vi "HXG2_FlowAir_STD51.vi"(0 "1\" Nozzle":bool, 1 "0.75\" Nozzle":bool, 2 "2.5inWC Sensor?":bool, 5 "1.25\" Nozzle":bool, 7 "1.5\" Nozzle":bool, 9 "Nozzle in Td °F":dbl, 11 "error in (no error)":errorcluster, 12 "Nozzle in %RH":dbl, 13 "Nozzle DP inWC":dbl, 14 "Pbarometric psi":dbl) -> (3 "CFM Nozzle":dbl, 4 "MaxSCFM":dbl, 6 "MinSCFM":dbl, 8 "Mdot (lbm/hr)":dbl, 10 "Rho per ASHRAE":dbl, 15 "error out":errorcluster)   [LabVIEW 2012]
doc: "This VI will calculate volumetric flow and provide the max and min flows that can be achieved with a particular nozzle combination."
panel:
  out "Pws Eqn":dbl
  out "Patm (psia)":dbl
  out "PabsUUT (inWC)":dbl
  out "All Psychrometric Calcs":sgl[](array[numeric])
  out "Pw":sgl
  out "W":sgl
  out "v":sgl
  out "ALPHA":sgl format="%#.3f"
  out "Ce 1":dbl[](array[numeric])
  out "Ce":dbl[](array[numeric])
  out "Re":dbl[](array[numeric])
  out "Y":sgl
  out "mu":sgl format="%#.6f"
  out "output variable":i16
  out "Pws":dbl
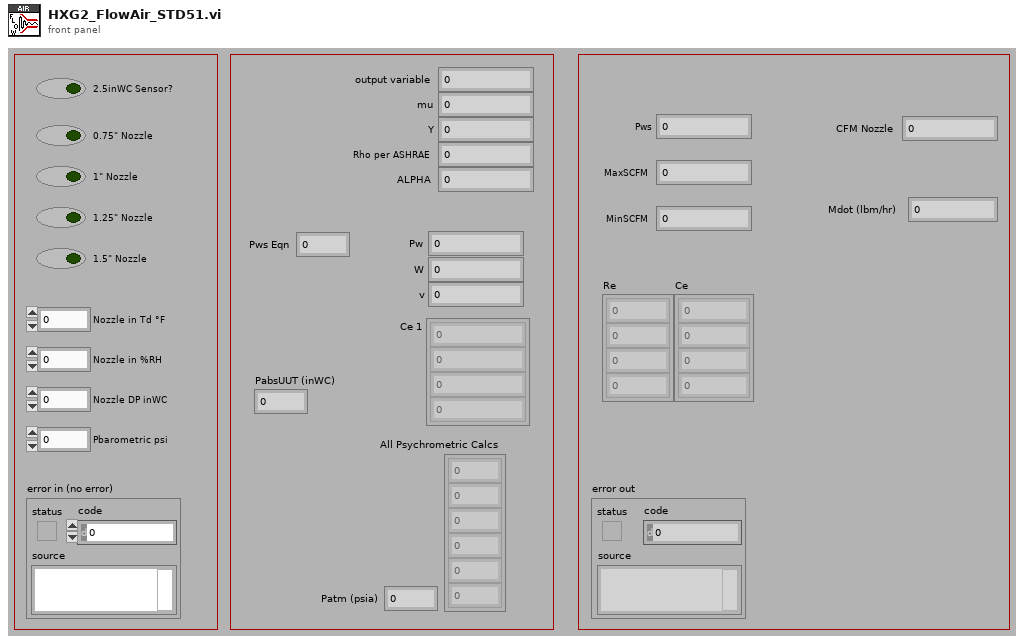
[diagram p1: front panel]
types:
  T1 = enum16{"Initial Values", "Closed Nozzle", "Iterate", "Recalc Re", "Done"}
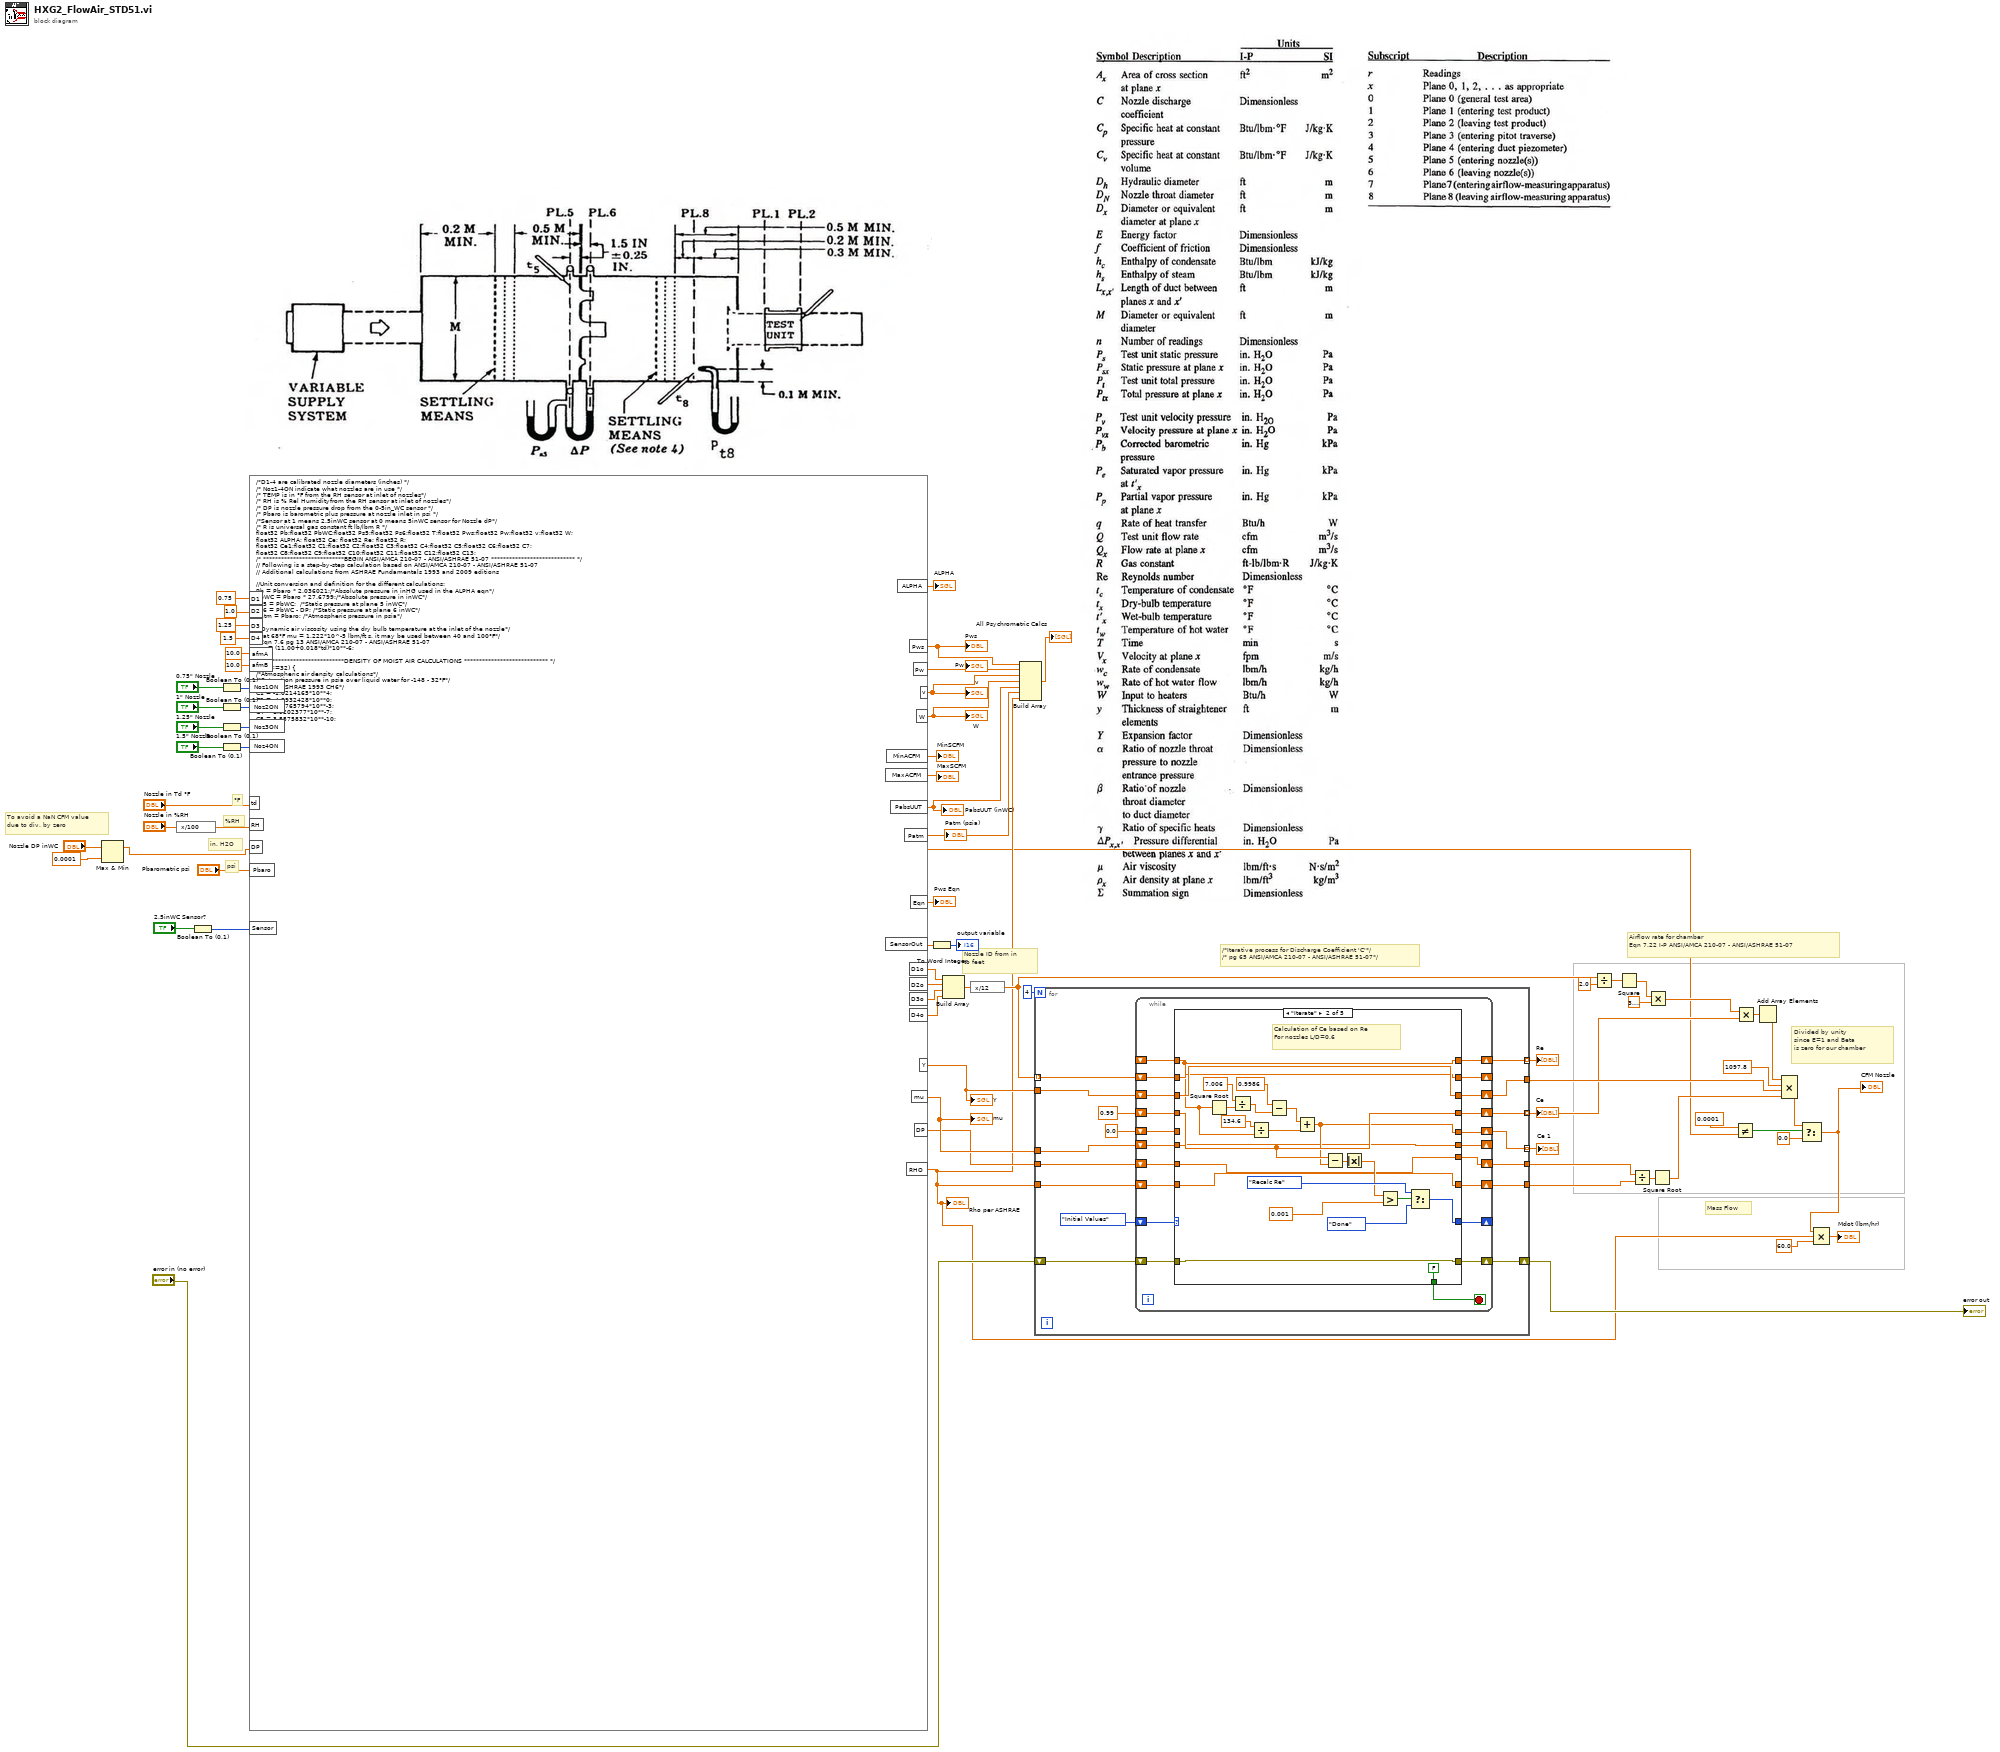
[diagram p0: block diagram]
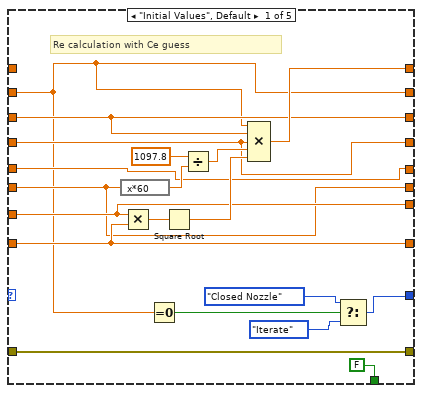
[diagram p2: hidden frame]
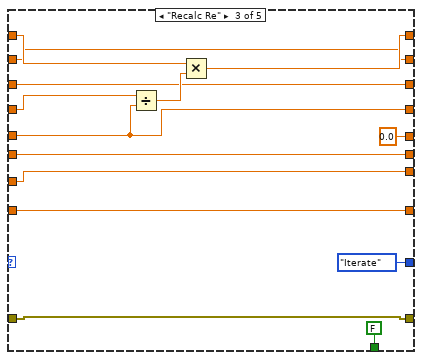
[diagram p3: hidden frame]
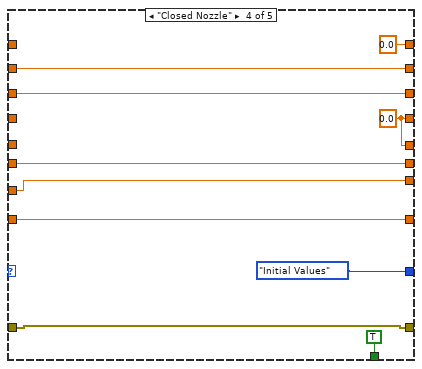
[diagram p4: hidden frame]
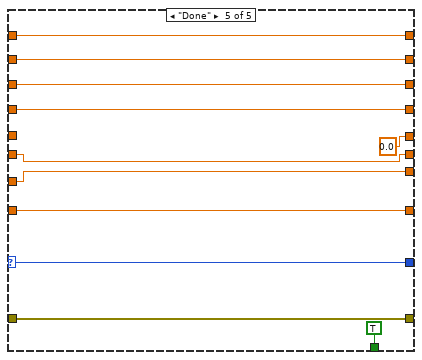
[diagram p5: hidden frame]
diagram:
  # "To avoid a NaN CFM value\ndue to div. by zero"
  # "Mass Flow"
  # "Nozzle ID from in\nto feet"
  # "Airflow rate for chamber\nEqn 7.22 I-P ANSI/AMCA 210-07 - ANSI/ASHRAE 51-07"
  # "Divided by unity\nsince E=1 and Beta\nis zero for our chamber"
  # "/*Iterative process for Discharge Coefficient 'C'*/\n/* pg 65 ANSI/AMCA 210-07 - ANSI/ASHRAE 51-07*/"
  # "in. H2O"
  # "%RH"
  # "°F"
  # "psi"
  n1 = Max & Min(x="Nozzle DP inWC", y=0.0001) -> (max(x,y)=w1:dbl)  [unwired: 1 out]
  n2 = expression code="x/100"("Nozzle in %RH") -> (w20:dbl)
  n3 = Boolean To (0,1)(Boolean="2.5inWC Sensor?") -> (0, 1=w53:i16)
  n4 = Boolean To (0,1)(Boolean="0.75\" Nozzle") -> (0, 1=w65:i16)
  n5 = Boolean To (0,1)(Boolean="1\" Nozzle") -> (0, 1=w67:i16)
  n6 = Boolean To (0,1)(Boolean="1.25\" Nozzle") -> (0, 1=w68:i16)
  n7 = Boolean To (0,1)(Boolean="1.5\" Nozzle") -> (0, 1=w66:i16)
  n8 = formula code="/*D1-4 are calibrated nozzle diameters (inches) */\n/* Noz1-4ON indicate what nozzles are in use */\n/* TEMP is in °F from the RH sensor at inlet of nozzles*/\n/* RH is % Rel Humidityfrom the RH sensor at inlet of nozzles*/\n/* DP is nozzle pressure drop from the 0-5in_WC sensor */\n/* Pbaro is barometric plus pressure at nozzle inlet in psi */ \n/*Sensor at 1 means 2.5inWC sensor at 0 means 5inWC sensor for Nozzle dP*/\n/* R is universal gas constant ft lb/lbm R */\nfloat32 Pb;float32 PbWC;float32 Ps5;float32 Ps6;float32 T;float32 Pws;float32 Pw;float32 v;float32 W;\nfloat32 ALPHA; float32 Ce; float32 Re; float32 R;\nfloat32 Ce1;float32 C1;float32 C2;float32 C3;float32 C4;float32 C5;float32 C6;float32 C7;\nfloat32 C8;float32 C9;float32 C10;float32 C11;float32 C12;float32 C13;\n/* ***************************BEGIN ANSI/AMCA 210-07 - ANSI/ASHRAE 51-07 **************************** */\n// Following is a step-by-step calculation based on ANSI/AMCA 210-07 - ANSI/ASHRAE 51-07\n// Additional calculations from ASHRAE Fundamentals 1993 and 2009 editions\n\n//Unit conversion and definition for the different calculations:\nPb = Pbaro * 2.036021;/*Absolute pressure in inHG used in the ALPHA eqn*/\nPbWC = Pbaro * 27.6799;/*Absolute pressure in inWC*/\nPs5 = PbWC;  /*Static pressure at plane 5 inWC*/\nPs6 = PbWC - DP; /*Static pressure at plane 6 inWC*/\nPatm = Pbaro; /*Atmospheric pressure in psia*/\n\n/*Dynamic air viscosity using the dry bulb temperature at the inlet of the nozzle*/\n/* at 68°F mu = 1.222*10^-5 lbm/ft s, it may be used between 40 and 100°F*/\n//Eqn 7.6 pg 13 ANSI/AMCA 210-07 - ANSI/ASHRAE 51-07\nmu = (11.00+0.018*td)*10**-6;\n\n/* ***************************DENSITY OF MOIST AIR CALCULATIONS **************************** */\nif (td<=32) {\n/*Atmospheric air density calculations*/\n/*Saturation pressure in psia over liquid water for -148 - 32°F*/\n/*Eqn 4 ASHRAE 1993 CH6*/\nC1 = -1.0214165*10**4;\nC2 = -4.8932428*10**0;\nC3 = -5.3765794*10**-3;\nC4 = 1.9202377*10**-7;\nC5 = 3.5575832*10**-10;\nC6 = -9.0344688*10**-14;\nC7 = 4.1635019;\nT = td+459.67;\nPws = exp(C1/T + C2 + C3*T + C4*T**2 + C5*T**3 + C6*T**4 + C7*ln(T)); /*psia*/\nEqn = 1;\n}\nelse{\n/*Atmospheric air density calculations*/\n/*Saturation pressure in psia over liquid water for 32-392°F*/\n/*Eqn 4 ASHRAE 1993 CH6*/\nC8 = -1.0440397*10**4;\nC9 = -1.1294650*10**1;\nC10 = -2.7022355*10**-2;\nC11= 1.2890360*10**-5;\nC12 = -2.4780681*10**-9;\nC13 = 6.5459673;\nT = td+459.67;\nPws = exp(C8/T + C9 + C10*T + C11*T**2 + C12*T**3 +C13*ln(T)); /*psia*/\nEqn = 2;\n}\n/*Partial pressure of water vapor (Pw=Pe)*/\n/*Eqn 22 ASHRAE 1993 CH6*/\nPw = RH*Pws; /*psia*/\n\n/*Humidity ratio W*/\n/*Total pressure of moist air in psi is Pbaro*/\n/*Eqn 23 ASHRAE 2009 CH1*/\nW = 0.621945*(Pw/(Pbaro-Pw));\n\n/*Specific volume of moist air mixture v*/\n/*Eqn 28 ASHRAE 2009 CH1*/\nv = 0.370486*T*(1+1.607858*W)/Pbaro; /*cft/lbs of dry air*/\n\n/*Density of Moist Air*/\n/*Eqn 11 ASHRAE 1993 CH6*/\nRHO = (1/v)*(1+W);\n/* ***********************END DENSITY OF MOIST AIR CALCULATIONS **************************** */\n\n/*Alpha ratio: The ratio of absolute nozzle exit pressure to absolute approach pressure*/\n//Eqn 7.12 pg14 ANSI/AMCA 210-07 - ANSI/ASHRAE 51-07\nR = 53.35;\n/* ALPHAB = (Ps6 + 13.595*Pb)/(Ps5 + 13.595*Pb); OLD FORMULA WITH PRESSURES AT EACH PLANE*/\nALPHA = 1-((5.2014*DP)/(RHO*R*(td+459.67)));\n\n/* Beta ratio: The ration of nozzle exit diameter D6 to approach duct diameter D5*/\n/* For a chamber approach Beta may be taken as zero*/\n\n/*Expansion Factor Y*/\nY = sqrt( (1.4/(1.4-1)) * (ALPHA**(2/1.4)) * ( (1-ALPHA**((1.4-1)/1.4)) / (1-ALPHA)));\n\n/*Energy Factor (E): Maybe determined by measuring velocity pressures  upstream of the nozzle*/\n/* Sufficient accurracy for this standard maybe obtained by setting E = 1.0 for chamber approach*/\n/* and E = 1.043 for duct approach.  Since E=1.0 it will be omitted in all calculations, it is a multiplier*/\n\n//Constant that will be sent to iterative solver for discharge coefficient calculations\nD1o = D1*Noz1ON;\nD2o = D2*Noz2ON;\nD3o = D3*Noz3ON;\nD4o = D4*Noz4ON;\n/* ***************************END ANSI/AMCA 210-07 - ANSI/ASHRAE 51-07 **************************** */\n\n//Chamber specific calculations\nSensorOut = Sensor;\n/*For 2.5inWC sensor*/\n/*Max and Min flow calculated from 2.45 and 0.35inWC limit pressures*/\n\nif(Sensor==1) {\nMaxACFM = Noz1ON*18.5 + Noz2ON*33 + Noz3ON*51.7 + Noz4ON*74.7;\nMinACFM = Noz1ON*6.9 + Noz2ON*12.3 + Noz3ON*19.3 + Noz4ON*27.9;\n}\n/*For 5inWC sensor*/\nelse {\nMaxACFM = Noz1ON*25.11 + Noz2ON*44.8 + Noz3ON*70.17 + Noz4ON*101.24;\nMinACFM = Noz1ON*11.8 + Noz2ON*21.0 + Noz3ON*32.9 + Noz4ON*47.5;\n}\n\n/* **************************************************************************** */"("D2"=1.0 ("input variable"), "D4"=1.5 ("input variable"), "D1"=0.75 ("input variable"), "D3"=1.25 ("input variable"), "DP"=w1, "Pbaro"="Pbarometric psi", "td"="Nozzle in Td °F", "RH"=w20, "afmA"=10.0 ("input variable"), "afmB"=10.0 ("input variable"), "Noz1ON"=w65, "Noz2ON"=w67, "Noz3ON"=w68, "Noz4ON"=w66, "Sensor"=w53) -> ("v"=w17:sgl, "Pws"=w19:sgl, "RHO"=w10:dbl, "ALPHA"=→"ALPHA":sgl, "MaxACFM"=→"MaxSCFM":dbl, "MinACFM"=→"MinSCFM":dbl, "SensorOut"=w51:dbl, "mu"=w50:dbl, "Y"=w44:dbl, "DP"=w43:dbl, "D1o"=w49:dbl, "D2o"=w48:dbl, "D3o"=w47:dbl, "D4o"=w46:dbl, "W"=w16:sgl, "Pw"=w18:sgl, "PabsUUT"=w12:dbl, "Patm"=w11:dbl, "Eqn"=→"Pws Eqn":dbl)
  "Pws" <- w19
  "Rho per ASHRAE" <- w10
  "mu" <- w50
  "Y" <- w44
  "v" <- w17
  "W" <- w16
  "Pw" <- w18
  "PabsUUT (inWC)" <- w12
  "Patm (psia)" <- w11
  n9 = To Word Integer(number=w51) -> (16bit integer=→"output variable":i16)
  n10 = Build Array(w49, w48, w47, w46) -> (w24:dbl[])
  n11 = expression code="x/12"(w24) -> (w23:dbl[])
  n12 = Build Array(w19, w18, w17, w16, w12, w11, w10) -> (→"All Psychrometric Calcs":dbl[])
  n13 = for {
    N: 4 -> [_]
    tunnel: w50 -> [w87]
    tunnel: w23 -> [w85] mode=indexing
    tunnel: w44 -> [w84]
    tunnel: w43 -> [w83]
    tunnel: w10 -> [w82]
    tunnel: [w81] -> w42 mode=indexing
    tunnel: [w80] -> w30 mode=indexing
    tunnel: [w78] -> w41 mode=indexing
    shift-right: [w76] -> w35
    shift-left: "error in (no error)" -> [w77]
    tunnel: [w75] -> w34
    tunnel: [w74] -> w27
    tunnel: [w73] -> w33
    n14 = while {
      shift-right: [w108] -> _
      shift-left: T1."Initial Values" ("Enum") -> [w109]
      shift-right: [w98] -> w80
      shift-left: 0.99 ("x") -> [w106]
      shift-right: [w100] -> w81
      shift-left: _ -> [w99]
      shift-right: [w96] -> w78
      shift-left: 0.0 ("x") -> [w97]
      shift-right: [w95] -> w73
      shift-left: w82 -> [w101]
      shift-right: [w94] -> w74
      shift-left: w83 -> [w102]
      shift-right: [w93] -> _
      shift-left: w87 -> [w107]
      shift-right: [w92] -> w75
      shift-left: w84 -> [w103]
      shift-right: [w91] -> _
      shift-left: w85 -> [w104]
      shift-right: [w89] -> w76
      shift-left: w77 -> [w90]
      stop <- w105 stop-if-true
      n15 = case shown="\"Iterate\"" w109 {
        selector: w109 -> [_ _ _ _ w184]
        tunnel: [w120 w143 T1."Iterate" ("Enum") T1."Initial Values" ("Enum") w184] -> w108
        tunnel: w107 -> [w113 w133 w156 w170 w180]
        tunnel: w106 -> [w116 w139 w165 _ w186]
        tunnel: [FALSE FALSE FALSE TRUE TRUE] -> w105
        tunnel: w104 -> [w110 w131 w154 w168 w178]
        tunnel: w103 -> [w112 w132 w155 w169 w179]
        tunnel: w102 -> [w114 w134 w157 w171 w181]
        tunnel: w101 -> [w115 w135 w158 w172 w182]
        tunnel: [w122 w130 w162 0.0 w187] -> w100
        tunnel: w99 -> [_ w130 w163 _ w187]
        tunnel: [w116 w139 w160 w174 w186] -> w98
        tunnel: [w117 w138 0.0 ("x") w174 0.0 ("x")] -> w96
        tunnel: w97 -> [w117 _ w160 _ _]
        tunnel: [w115 w135 w158 w172 w182] -> w95
        tunnel: [w114 w134 w157 w171 w181] -> w94
        tunnel: [w113 w133 w156 w170 w180] -> w93
        tunnel: [w112 w132 w155 w169 w179] -> w92
        tunnel: [w110 w131 w154 w168 w178] -> w91
        tunnel: w90 -> [w111 w129 w153 w167 w177]
        tunnel: [w111 w129 w153 w167 w177] -> w89
        frame "Initial Values", Default {
          # "Re calculation with Ce guess"
          n16 = expression code="x*60"(w113) -> (w127:dbl)
          n17 = Multiply(x=w114, y=w115) -> (x*y=w124:dbl)
          n18 = Equal To 0?(x=w110) -> (x = 0?=w121:bool)
          n19 = Square Root(x=w124) -> (sqrt(x)=w123:dbl)
          n20 = Divide(x=1097.8, y=w127) -> (x/y=w126:dbl)
          n21 = Compound Arithmetic op=MULTIPLY(w110, w112, w116, w126, w123) -> (w122:dbl)
          n22 = Select(t=T1."Closed Nozzle" ("Enum"), s=w121, f=T1."Iterate" ("Enum")) -> (s? t:f=w120:T1)
        }
        frame "Iterate" {
          # "Calculation of Ce based on Re\nFor nozzles L/D=0.6"
          n23 = Square Root(x=w130) -> (sqrt(x)=w147:dbl)
          n24 = Divide(x=7.006, y=w147) -> (x/y=w149:dbl)
          n25 = Divide(x=134.6, y=w130) -> (x/y=w146:dbl)
          n26 = Subtract(x=0.9986, y=w149) -> (x-y=w150:dbl)
          n27 = Add(x=w150, y=w146) -> (x+y=w138:dbl)
          n28 = Subtract(x=w139, y=w138) -> (x-y=w137:dbl)
          n29 = Absolute Value(x=w137) -> (abs(x)=w136:dbl)
          n30 = Greater?(x=w136, y=0.001) -> (0:w145:bool)
          n31 = Select(t=T1."Recalc Re" ("Enum"), s=w145, f=T1."Done" ("Enum")) -> (s? t:f=w143:T1)
        }
        frame "Recalc Re" {
          n32 = Divide(x=w165, y=w160) -> (x/y=w164:dbl)
          n33 = Multiply(x=w163, y=w164) -> (x*y=w162:dbl)
        }
        frame "Closed Nozzle" {
          w174 = 0.0 ("x")
        }
        frame "Done" {
        }
      }
    }
  }
  "error out" <- w35
  "Re" <- w42
  "Ce" <- w30
  "Ce 1" <- w41
  n34 = Divide(x=w23, y=2.0 ("x")) -> (x/y=w39:dbl[])
  n35 = Square(x=w39) -> (x^2=w37:dbl[])
  n36 = Divide(x=w27, y=w33) -> (x/y=w32:dbl)
  n37 = Multiply(x=w37, y=3.141592653589793) -> (x*y=w31:dbl[])
  n38 = Square Root(x=w32) -> (sqrt(x)=w26:dbl)
  n39 = Not Equal?(x=0.0001, y=w1) -> (x != y?=w6:bool)
  n40 = Multiply(x=w31, y=w30) -> (x*y=w29:dbl[])
  n41 = Add Array Elements(numeric array=w29) -> (sum=w25:dbl)
  n42 = Compound Arithmetic op=MULTIPLY(w25, 1097.8 ("x"), w34, w26) -> (w4:dbl)
  n43 = Select(t=w4, s=w6, f=0.0) -> (s? t:f=w3:dbl)
  "CFM Nozzle" <- w3
  n44 = Compound Arithmetic op=MULTIPLY(w3, w10, 60.0 ("value")) -> (→"Mdot (lbm/hr)":dbl)
